vi "header_data.vi"(8 "error in":errorcluster, 11 "midi-file in":refnum<class "midi-file.lvclass">) -> (0 "error out":errorcluster, 3 "midi-file out":refnum<class "midi-file.lvclass">)   [LabVIEW 2020, in "midi-file.lvclass"]
uses:
  midi-file.lvclass
  file_format.ctl
  midi-file.lvclass/midi-file.ctl
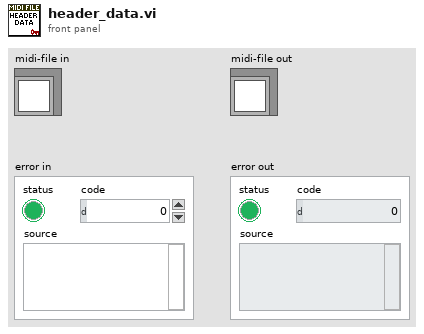
[diagram p1: front panel]
types:
  T1 = typedef "midi-file.lvclass/file_format.ctl" = enum16{"single track file format", "multiple track file format", "multiple song file format"}
  T2 = cluster{"header length":i32, "format":T1, "number of tracks":i16, "division":i16}
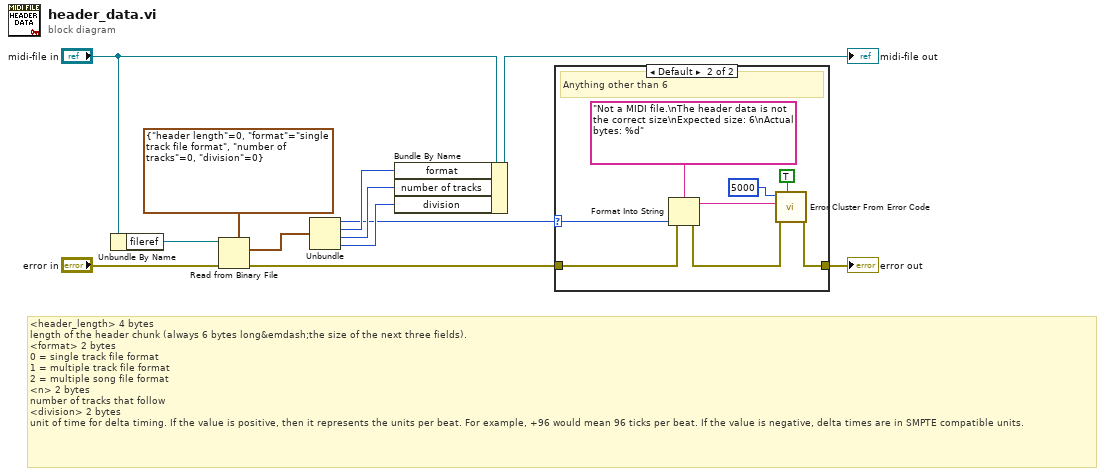
[diagram p0: block diagram]
diagram:
  # "<header_length> 4 bytes\nlength of the header chunk (always 6 bytes long&emdash;the size of the next three fields).\n<format> 2 bytes\n0 = single track file format\n1 = multiple track file format\n2 = multiple song file format\n<n> 2 bytes\nnumber of tracks that follow\n<division> 2 bytes\nunit of time for delta timing. If the value is positive, then it represents the units per beat. For example, +96 would mean 96 ticks per beat. If the value is negative, delta times are in SMPTE compatible units."
  n1 = Unbundle By Name("midi-file in") -> ("fileref"=w12:refnum<file>)
  n2 = Read from Binary File(5:T2 {"header length"=0, "format"=enum."single track file format", "number of tracks"=0, "division"=0}, 8:"error in", 11:w12) -> (0:w1:errorcluster, 2:w8:T2)  [unwired: 3 in, 2 out]
  n3 = Unbundle(w8) -> ("header length"=w3:i32, "format"=w7:T1, "number of tracks"=w6:i16, "division"=w5:i16)
  n4 = Bundle By Name(cluster="midi-file in", "format"=w7, "number of tracks"=w6, "division"=w5) -> (→"midi-file out":refnum<class "midi-file.lvclass">)
  n5 = case shown="Default" w3 {
    selector: w3 -> [_ w14]
    tunnel: w1 -> [w13 w16]
    tunnel: [w13 w15] -> w2
    frame 6 {
      # "6 is the expected number of bytes"
    }
    frame Default {
      # "Anything other than 6"
      n6 = Format Into String(format string="Not a MIDI file.\nThe header data is not the correct size\nExpected size: 6\nActual bytes: %d" ("error message (\"\")"), error in=w16, w14) -> (resulting string=w18:string, error out=w17:errorcluster)  [unwired: 1 in]
      n7 = call <vilib>:"Error Cluster From Error Code.vi"("show call chain? (False)"=TRUE, "error in (no error)"=w17, "error message (\"\")"=w18, "error code (0)"=5000) -> ("error out"=w15:errorcluster)  [unwired: 5 in]
    }
  }
  "error out" <- w2
